vi "VISA Event.vi"(8 "Error In":errorcluster, 9 "Test Duration (ms)":u32=10000, 10 "Timeout (ms)":u32=10000, 11 "VISA resource":refnum<visa-resource-name>="COM3") -> (0 "Error Out":errorcluster, 1 "Instrument Data(Random)":string, 3 "Correct Response Rate %":dbl(slide) scale=0.0..100.0, 4 "No of Reponse":i32, 5 "No of False Polling":i32)   [LabVIEW 2015]
uses:
  <vilib>/Instr/_visa.llb/Select Event Type.ctl
  <vilib>/Instr/_visa.llb/VISA Event Mechanism.ctl
  <vilib>/Instr/_visa.llb/VISA Configure Serial Port (Instr).vi
panel:
  in  "STOP":bool
  # "Event"
  # "x 100"
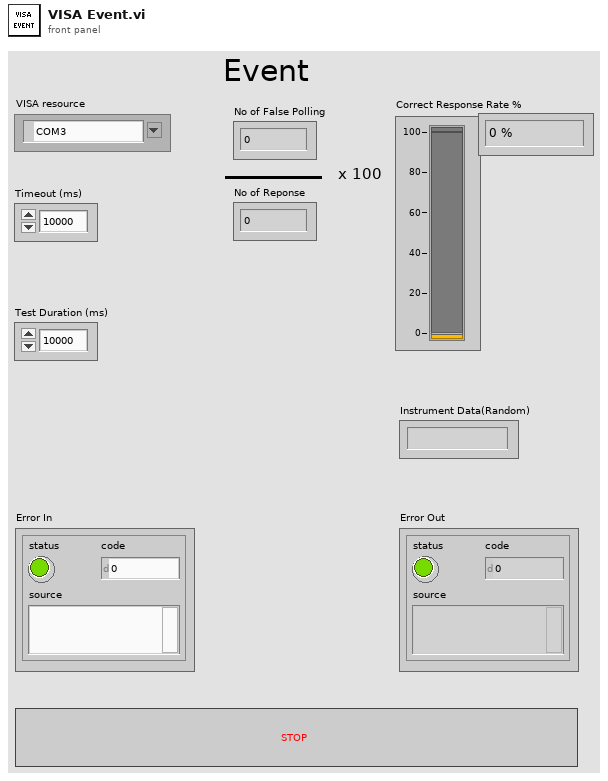
[diagram p1: front panel]
types:
  T1 = typedef "VISA Event Mechanism.ctl" = u16
  T2 = typedef "Select Event Type.ctl" = u32
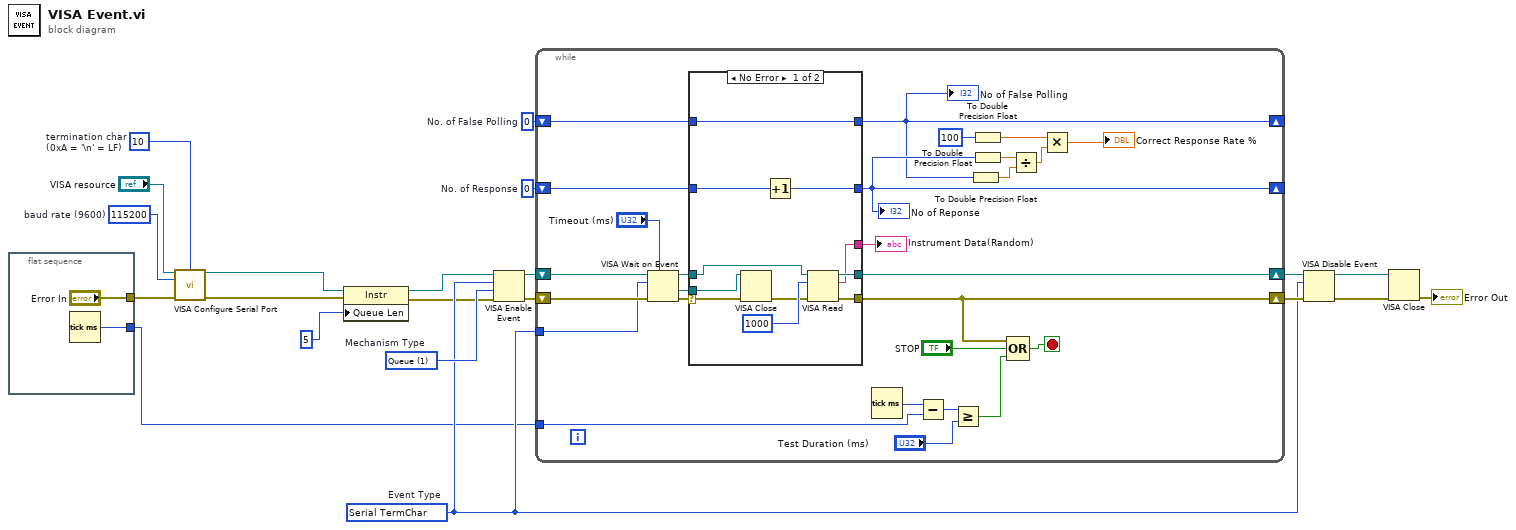
[diagram p0: block diagram]
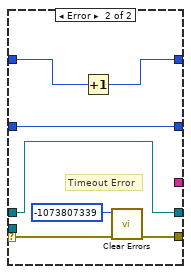
[diagram p2: hidden frame]
diagram:
  w4 = 0  # No. of False Polling
  w5 = 0  # No. of Response
  w12 = T1 1 items=["Queue"=1]  # Mechanism Type
  w9 = T2 1073684516 items=["Service Request"=1073684491, "Trigger"=3221168138, "Clear"=1073684493, "VXI Signal"=1073684512, "VXI/VME Interrupt"=3221168161, "VXI/VME Sysfail"=1073684509, "VXI/VME Sysreset"=1073684510, "GPIB CIC"=1073684498, "GPIB Talk"=1073684499, "GPIB Listen"=1073684500, "PXI Interrupt"=1073684514, "Serial Break"=1073684515, "Serial TermChar"=1073684516, "Serial CTS"=1073684521, "Serial DSR"=1073684522, "Serial DCD"=1073684524, "Serial RI"=1073684526, "Serial Character"=1073684533, "USB Interrupt"=1073684535, "All Enabled"=1073709055]  # Event Type
  w20 = u8 10  # termination char (0xA = '\n' = LF)
  w21 = u32 115200  # baud rate (9600)
  n1 = flat-sequence {
    tunnel: [w23] -> w1
    tunnel: ["Error In"] -> w3
    frame #0 {
      n2 = Tick Count (ms)() -> (millisecond timer value=w23:u32)
    }
  }
  n3 = call-poly "VISA Configure Serial Port"("VISA resource name"="VISA resource", "termination char\n(0xA = '\\n' = LF)"=w20, "baud rate (9600)"=w21, "error in (no error)"=w3) -> ("VISA resource name out"=w15:refnum<visa-resource-name>, "error out"=w16:errorcluster)  [unwired: 10 in]
  n4 = property class="Instr"(reference=w15, error in=w16, "Queue Len"=u32 5 ("i")) -> (reference out=w6:refnum<visa-resource-name>, error out=w7:errorcluster)
  n5 = VISA Enable Event(8:w7, 9:w12, 10:w9, 11:w6) -> (0:w11:errorcluster, 3:w10:refnum<visa-resource-name>)
  n6 = while {
    shift-right: [w45] -> w14
    shift-left: w11 -> [w50]
    tunnel: w9 -> [w43]
    shift-right: [w44] -> w13
    shift-left: w10 -> [w46]
    shift-right: [w30] -> _
    shift-left: w5 -> [w37]
    shift-right: [w29] -> _
    shift-left: w4 -> [w38]
    tunnel: w1 -> [w27]
    stop <- w41 stop-if-true
    n7 = VISA Wait on Event(7:"Timeout (ms)", 8:w50, 10:w43, 11:w46) -> (0:w47:errorcluster, 1:w48:refnum<visa-resource-name>, 3:w42:refnum<visa-resource-name>)  [unwired: 1 in, 1 out]
    n8 = case shown="No Error" w47 {
      selector: w47 -> [w60 w68]
      tunnel: w48 -> [w61 _]
      tunnel: [w59 w66] -> w45
      tunnel: [w58 w67] -> w44
      tunnel: w42 -> [w57 w67]
      tunnel: [w54 _] -> w39
      tunnel: w38 -> [w53 w64]
      tunnel: [w53 w62] -> w29
      tunnel: w37 -> [w52 w63]
      tunnel: [w51 w63] -> w30
      frame No Error {
        n9 = VISA Close(VISA resource name=w61, error in (no error)=w60) -> (error out=w55:errorcluster)
        n10 = Increment(x=w52) -> (x+1=w51:i32)
        n11 = VISA Read(VISA resource name=w57, byte count=u32 1000, error in (no error)=w55) -> (VISA resource name out=w58:refnum<visa-resource-name>, read buffer=w54:string, error out=w59:errorcluster)  [unwired: 1 out]
      }
      frame Error {
        # "Timeout Error"
        n12 = Increment(x=w64) -> (x+1=w62:i32)
        n13 = call <vilib>:"Clear Errors.vi"("error in (no error)"=w68, "specific error code to clear (0: all)"=-1073807339) -> ("error out"=w66:errorcluster)  [unwired: 4 in, 1 out]
      }
    }
    "Instrument Data(Random)" <- w39
    "No of Reponse" <- w30
    "No of False Polling" <- w29
    n14 = Tick Count (ms)() -> (millisecond timer value=w28:u32)
    n15 = Subtract(x=w28, y=w27) -> (x-y=w26:u32)
    n16 = Greater Or Equal?(x=w26, y="Test Duration (ms)") -> (x >= y?=w24:bool)
    n17 = To Double Precision Float(number=w29) -> (double precision float=w32:dbl)
    n18 = To Double Precision Float(number=100 ("x")) -> (double precision float=w34:dbl)
    n19 = To Double Precision Float(number=w30) -> (double precision float=w31:dbl)
    n20 = Compound Arithmetic op=OR(w45, "STOP", w24) -> (w41:bool)
    n21 = Divide(x=w31, y=w32) -> (x/y=w35:dbl)
    n22 = Multiply(x=w34, y=w35) -> (x*y=→"Correct Response Rate %":dbl)
  }
  n23 = VISA Disable Event(8:w14, 10:w9, 11:w13) -> (0:w18:errorcluster, 3:w17:refnum<visa-resource-name>)  [unwired: 1 in]
  n24 = VISA Close(VISA resource name=w17, error in (no error)=w18) -> (error out=→"Error Out":errorcluster)
